vi "GeoData.vi"() -> ()   [LabVIEW 2017] (continued)
Davison County\tH1\n57235\t46037\tFlorence\tSD\tDay County\tH1\n57239\t46037\tGrenville\tSD\tDay County\tH1\n57434\t46037\tConde\tSD\tDay County\tH1\n57273\t46037\tWaubay\tSD\tDay County\tH1\n57454\t46037\tLangford\tSD\tDay County\tH1\n57232\t46037\tEden\tSD\tDay County\tH1\n57272\t46037\tWallace\tSD\tDay County\tH1\n57422\t46037\tAndover\tSD\tDay County\tH1\n57274\t46037\tWebster\tSD\tDay County\tH1\n57445\t46037\tGroton\tSD\tDay County\tH1\n57219\t46037\tBristol\tSD\tDay County\tH1\n57468\t46037\tPierpont\tSD\tDay County\tH1\n57256\t46037\tOrtley\tSD\tDay County\tH1\n57261\t46037\tRoslyn\tSD\tDay County\tH1\n57234\t46039\tEstelline\tSD\tDeuel County\tH1\n57238\t46039\tGoodwin\tSD\tDeuel County\tH1\n57268\t46039\tToronto\tSD\tDeuel County\tH1\n57265\t46039\tStrandburg\tSD\tDeuel County\tH1\n57213\t46039\tAstoria\tSD\tDeuel County\tH1\n57226\t46039\tClear lake\tSD\tDeuel County\tH1\n57223\t46039\tCastlewood\tSD\tDeuel County\tH1\n57237\t46039\tGary\tSD\tDeuel County\tH1\n57259\t46039\tRevillo\tSD\tDeuel County\tH1\n57218\t46039\tBrandt\tSD\tDeuel County\tH1\n57652\t46041\tRidgeview\tSD\tDewey County\tH1\n57657\t46041\tTrail city\tSD\tDewey County\tH1\n57633\t46041\tIsabel\tSD\tDewey County\tH1\n57630\t46041\tGlencross\tSD\tDewey County\tH1\n57636\t46041\tLantry\tSD\tDewey County\tH1\n57656\t46041\tTimber lake\tSD\tDewey County\tH1\n57625\t46041\tEagle butte\tSD\tDewey County\tH1\n57661\t46041\tWhitehorse\tSD\tDewey County\tH1\n57344\t46043\tHarrison\tSD\tDouglas County\tH1\n57313\t46043\tArmour\tSD\tDouglas County\tH1\n57369\t46043\tPlatte\tSD\tDouglas County\tH1\n57328\t46043\tCorsica\tSD\tDouglas County\tH1\n57331\t46043\tDimock\tSD\tDouglas County\tH1\n57375\t46043\tStickney\tSD\tDouglas County\tH1\n57330\t46043\tDelmont\tSD\tDouglas County\tH1\n57364\t46043\tNew holland\tSD\tDouglas County\tH1\n57366\t46043\tParkston\tSD\tDouglas County\tH1\n57342\t46043\tGeddes\tSD\tDouglas County\tH1\n57451\t46045\tIpswich\tSD\tEdmunds County\tH1\n57428\t46045\tBowdle\tSD\tEdmunds County\tH1\n57460\t46045\tMansfield\tSD\tEdmunds County\tH1\n57471\t46045\tRoscoe\tSD\tEdmunds County\tH1\n57481\t46045\tWestport\tSD\tEdmunds County\tH1\n57448\t46045\tHosmer\tSD\tEdmunds County\tH1\n57435\t46045\tCresbard\tSD\tEdmunds County\tH1\n57475\t46045\tTolstoy\tSD\tEdmunds County\tH1\n57456\t46045\tLeola\tSD\tEdmunds County\tH1\n57466\t46045\tOnaka\tSD\tEdmunds County\tH1\n57722\t46047\tBuffalo gap\tSD\tFall River County\tH1\n57747\t46047\tHot springs\tSD\tFall River County\tH1\n57782\t46047\tSmithwick\tSD\tFall River County\tH1\n57735\t46047\tEdgemont\tSD\tFall River County\tH1\n57766\t46047\tOral\tSD\tFall River County\tH1\n57763\t46047\tOelrichs\tSD\tFall River County\tH1\n57460\t46049\tMansfield\tSD\tFaulk County\tH1\n57438\t46049\tFaulkton\tSD\tFaulk County\tH1\n57424\t46049\tAshton\tSD\tFaulk County\tH1\n57469\t46049\tRedfield\tSD\tFaulk County\tH1\n57470\t46049\tRockham\tSD\tFaulk County\tH1\n57435\t46049\tCresbard\tSD\tFaulk County\tH1\n57467\t46049\tOrient\tSD\tFaulk County\tH1\n57473\t46049\tSeneca\tSD\tFaulk County\tH1\n57465\t46049\tNorthville\tSD\tFaulk County\tH1\n57345\t46049\tHighmore\tSD\tFaulk County\tH1\n57466\t46049\tOnaka\tSD\tFaulk County\tH1\n57252\t46051\tMilbank\tSD\tGrant County\tH1\n57279\t46051\tWilmot\tSD\tGrant County\tH1\n57216\t46051\tBig stone city\tSD\tGrant County\tH1\n57273\t46051\tWaubay\tSD\tGrant County\tH1\n57227\t46051\tCorona\tSD\tGrant County\tH1\n57238\t46051\tGoodwin\tSD\tGrant County\tH1\n57263\t46051\tSouth shore\tSD\tGrant County\tH1\n57265\t46051\tStrandburg\tSD\tGrant County\tH1\n57266\t46051\tSummit\tSD\tGrant County\tH1\n57246\t46051\tLabolt\tSD\tGrant County\tH1\n57269\t46051\tTwin brooks\tSD\tGrant County\tH1\n57251\t46051\tMarvin\tSD\tGrant County\tH1\n57264\t46051\tStockholm\tSD\tGrant County\tH1\n57256\t46051\tOrtley\tSD\tGrant County\tH1\n57259\t46051\tRevillo\tSD\tGrant County\tH1\n57529\t46053\tDallas\tSD\tGregory County\tH1\n57538\t46053\tHerrick\tSD\tGregory County\tH1\n57317\t46053\tBonesteel\tSD\tGregory County\tH1\n57335\t46053\tFairfax\tSD\tGregory County\tH1\n57523\t46053\tBurke\tSD\tGregory County\tH1\n57571\t46053\tSaint charles\tSD\tGregory County\tH1\n57533\t46053\tGregory\tSD\tGregory County\tH1\n57552\t46055\tMidland\tSD\tHaakon County\tH1\n57567\t46055\tPhilip\tSD\tHaakon County\tH1\n57775\t46055\tQuinn\tSD\tHaakon County\tH1\n57543\t46055\tKadoka\tSD\tHaakon County\tH1\n57553\t46055\tMilesville\tSD\tHaakon County\tH1\n57234\t46057\tEstelline\tSD\tHamlin County\tH1\n57233\t46057\tErwin\tSD\tHamlin County\tH1\n57221\t46057\tBryant\tSD\tHamlin County\tH1\n57238\t46057\tGoodwin\tSD\tHamlin County\tH1\n57212\t46057\tArlington\tSD\tHamlin County\tH1\n57271\t46057\tVienna\tSD\tHamlin County\tH1\n57242\t46057\tHazel\tSD\tHamlin County\tH1\n57241\t46057\tHayti\tSD\tHamlin County\tH1\n57248\t46057\tLake norden\tSD\tHamlin County\tH1\n57226\t46057\tClear lake\tSD\tHamlin County\tH1\n57201\t46057\tWatertown\tSD\tHamlin County\tH1\n57243\t46057\tHenry\tSD\tHamlin County\tH1\n57223\t46057\tCastlewood\tSD\tHamlin County\tH1\n57476\t46059\tTulare\tSD\tHand County\tH1\n57469\t46059\tRedfield\tSD\tHand County\tH1\n57470\t46059\tRockham\tSD\tHand County\tH1\n57362\t46059\tMiller\tSD\tHand County\tH1\n57381\t46059\tWessington\tSD\tHand County\tH1\n57373\t46059\tSaint lawrence\tSD\tHand County\tH1\n57371\t46059\tRee heights\tSD\tHand County\tH1\n57467\t46059\tOrient\tSD\tHand County\tH1\n57382\t46059\tWessington springs\tSD\tHand County\tH1\n57345\t46059\tHighmore\tSD\tHand County\tH1\n57319\t46061\tBridgewater\tSD\tHanson County\tH1\n57340\t46061\tFulton\tSD\tHanson County\tH1\n57311\t46061\tAlexandria\tSD\tHanson County\tH1\n57334\t46061\tEthan\tSD\tHanson County\tH1\n57374\t46061\tSpencer\tSD\tHanson County\tH1\n57301\t46061\tMitchell\tSD\tHanson County\tH1\n57321\t46061\tCanova\tSD\tHanson County\tH1\n57332\t46061\tEmery\tSD\tHanson County\tH1\n57366\t46061\tParkston\tSD\tHanson County\tH1\n57760\t46063\tNewell\tSD\tHarding County\tH1\n57650\t46063\tRalph\tSD\tHarding County\tH1\n57755\t46063\tLudlow\tSD\tHarding County\tH1\n57651\t46063\tReva\tSD\tHarding County\tH1\n57717\t46063\tBelle fourche\tSD\tHarding County\tH1\n57720\t46063\tBuffalo\tSD\tHarding County\tH1\n57724\t46063\tCamp crook\tSD\tHarding County\tH1\n57649\t46063\tPrairie city\tSD\tHarding County\tH1\n57776\t46063\tRedig\tSD\tHarding County\tH1\n57501\t46065\tPierre\tSD\tHughes County\tH1\n57564\t46065\tOnida\tSD\tHughes County\tH1\n57536\t46065\tHarrold\tSD\tHughes County\tH1\n57522\t46065\tBlunt\tSD\tHughes County\tH1\n57319\t46067\tBridgewater\tSD\tHutchinson County\tH1\n57043\t46067\tMarion\tSD\tHutchinson County\tH1\n57354\t46067\tKaylor\tSD\tHutchinson County\tH1\n57059\t46067\tScotland\tSD\tHutchinson County\tH1\n57311\t46067\tAlexandria\tSD\tHutchinson County\tH1\n57334\t46067\tEthan\tSD\tHutchinson County\tH1\n57331\t46067\tDimock\tSD\tHutchinson County\tH1\n57052\t46067\tOlivet\tSD\tHutchinson County\tH1\n57029\t46067\tFreeman\tSD\tHutchinson County\tH1\n57330\t46067\tDelmont\tSD\tHutchinson County\tH1\n57045\t46067\tMenno\tSD\tHutchinson County\tH1\n57332\t46067\tEmery\tSD\tHutchinson County\tH1\n57376\t46067\tTripp\tSD\tHutchinson County\tH1\n57366\t46067\tParkston\tSD\tHutchinson County\tH1\n57540\t46069\tHolabird\tSD\tHyde County\tH1\n57346\t46069\tStephan\tSD\tHyde County\tH1\n57564\t46069\tOnida\tSD\tHyde County\tH1\n57345\t46069\tHighmore\tSD\tHyde County\tH1\n57536\t46069\tHarrold\tSD\tHyde County\tH1\n57577\t46071\tWanblee\tSD\tJackson County\tH1\n57567\t46071\tPhilip\tSD\tJackson County\tH1\n57521\t46071\tBelvidere\tSD\tJackson County\tH1\n57543\t46071\tKadoka\tSD\tJackson County\tH1\n57750\t46071\tInterior\tSD\tJackson County\tH1\n57547\t46071\tLong valley\tSD\tJackson County\tH1\n57312\t46073\tAlpena\tSD\tJerauld County\tH1\n57385\t46073\tWoonsocket\tSD\tJerauld County\tH1\n57382\t46073\tWessington springs\tSD\tJerauld County\tH1\n57355\t46073\tKimball\tSD\tJerauld County\tH1\n57531\t46075\tDraper\tSD\tJones County\tH1\n57559\t46075\tMurdo\tSD\tJones County\tH1\n57562\t46075\tOkaton\tSD\tJones County\tH1\n57231\t46077\tDe smet\tSD\tKingsbury County\tH1\n57233\t46077\tErwin\tSD\tKingsbury County\tH1\n57221\t46077\tBryant\tSD\tKingsbury County\tH1\n57051\t46077\tOldham\tSD\tKingsbury County\tH1\n57212\t46077\tArlington\tSD\tKingsbury County\tH1\n57248\t46077\tLake norden\tSD\tKingsbury County\tH1\n57054\t46077\tRamona\tSD\tKingsbury County\tH1\n57323\t46077\tCarthage\tSD\tKingsbury County\tH1\n57386\t46077\tYale\tSD\tKingsbury County\tH1\n57249\t46077\tLake preston\tSD\tKingsbury County\tH1\n57353\t46077\tIroquois\tSD\tKingsbury County\tH1\n57214\t46077\tBadger\tSD\tKingsbury County\tH1\n57048\t46079\tMontrose\tSD\tLake County\tH1\n57058\t46079\tSalem\tSD\tLake County\tH1\n57042\t46079\tMadison\tSD\tLake County\tH1\n57017\t46079\tColman\tSD\tLake County\tH1\n57051\t46079\tOldham\tSD\tLake County\tH1\n57212\t46079\tArlington\tSD\tLake County\tH1\n57076\t46079\tWinfred\tSD\tLake County\tH1\n57054\t46079\tRamona\tSD\tLake County\tH1\n57018\t46079\tColton\tSD\tLake County\tH1\n57016\t46079\tChester\tSD\tLake County\tH1\n57022\t46079\tDell rapids\tSD\tLake County\tH1\n57075\t46079\tWentworth\tSD\tLake County\tH1\n57057\t46079\tRutland\tSD\tLake County\tH1\n57071\t46079\tVolga\tSD\tLake County\tH1\n57050\t46079\tNunda\tSD\tLake County\tH1\n57779\t46081\tSaint onge\tSD\tLawrence County\tH1\n57785\t46081\tSturgis\tSD\tLawrence County\tH1\n57759\t46081\tNemo\tSD\tLawrence County\tH1\n57783\t46081\tSpearfish\tSD\tLawrence County\tH1\n57754\t46081\tLead\tSD\tLawrence County\tH1\n57717\t46081\tBelle fourche\tSD\tLawrence County\tH1\n57793\t46081\tWhitewood\tSD\tLawrence County\tH1\n57732\t46081\tDeadwood\tSD\tLawrence County\tH1\n57799\t46081\tSpearfish\tSD\tLawrence County\tH1\n57032\t46083\tHarrisburg\tSD\tLincoln County\tH1\n57021\t46083\tDavis\tSD\tLincoln County\tH1\n57106\t46083\tSioux falls\tSD\tLincoln County\tH1\n57014\t46083\tCenterville\tSD\tLincoln County\tH1\n57027\t46083\tFairview\tSD\tLincoln County\tH1\n57064\t46083\tTea\tSD\tLincoln County\tH1\n57108\t46083\tSioux falls\tSD\tLincoln County\tH1\n57034\t46083\tHudson\tSD\tLincoln County\tH1\n57039\t46083\tLennox\tSD\tLincoln County\tH1\n57077\t46083\tWorthing\tSD\tLincoln County\tH1\n57013\t46083\tCanton\tSD\tLincoln County\tH1\n57004\t46083\tBeresford\tSD\tLincoln County\tH1\n57104\t46083\tSioux falls\tSD\tLincoln County\tH1\n57001\t46083\tAlcester\tSD\tLincoln County\tH1\n57576\t46085\tVivian\tSD\tLyman County\tH1\n57568\t46085\tPresho\tSD\tLyman County\tH1\n57544\t46085\tKennebec\tSD\tLyman County\tH1\n57569\t46085\tReliance\tSD\tLyman County\tH1\n57548\t46085\tLower brule\tSD\tLyman County\tH1\n57533\t46085\tGregory\tSD\tLyman County\tH1\n57534\t46085\tHamill\tSD\tLyman County\tH1\n57365\t46085\tOacoma\tSD\tLyman County\tH1\n57048\t46087\tMontrose\tSD\tMcCook County\tH1\n57053\t46087\tParker\tSD\tMcCook County\tH1\n57058\t46087\tSalem\tSD\tMcCook County\tH1\n57042\t46087\tMadison\tSD\tMcCook County\tH1\n57319\t46087\tBridgewater\tSD\tMcCook County\tH1\n57043\t46087\tMarion\tSD\tMcCook County\tH1\n57012\t46087\tCanistota\tSD\tMcCook County\tH1\n57047\t46087\tMonroe\tSD\tMcCook County\tH1\n57374\t46087\tSpencer\tSD\tMcCook County\tH1\n57035\t46087\tHumboldt\tSD\tMcCook County\tH1\n57321\t46087\tCanova\tSD\tMcCook County\tH1\n57332\t46087\tEmery\tSD\tMcCook County\tH1\n57428\t46089\tBowdle\tSD\tMcPherson County\tH1\n57471\t46089\tRoscoe\tSD\tMcPherson County\tH1\n57481\t46089\tWestport\tSD\tMcPherson County\tH1\n57437\t46089\tEureka\tSD\tMcPherson County\tH1\n57448\t46089\tHosmer\tSD\tMcPherson County\tH1\n57456\t46089\tLeola\tSD\tMcPherson County\tH1\n57457\t46089\tLong lake\tSD\tMcPherson County\tH1\n57247\t46091\tLake city\tSD\tMarshall County\tH1\n57454\t46091\tLangford\tSD\tMarshall County\tH1\n57432\t46091\tClaremont\tSD\tMarshall County\tH1\n57232\t46091\tEden\tSD\tMarshall County\tH1\n57430\t46091\tBritton\tSD\tMarshall County\tH1\n57262\t46091\tSisseton\tSD\tMarshall County\tH1\n57270\t46091\tVeblen\tSD\tMarshall County\tH1\n57421\t46091\tAmherst\tSD\tMarshall County\tH1\n57787\t46093\tUnion center\tSD\tMeade County\tH1\n57767\t46093\tOwanka\tSD\tMeade County\tH1\n57788\t46093\tVale\tSD\tMeade County\tH1\n57785\t46093\tSturgis\tSD\tMeade County\tH1\n57748\t46093\tHowes\tSD\tMeade County\tH1\n57701\t46093\tRapid city\tSD\tMeade County\tH1\n57702\t46093\tRapid city\tSD\tMeade County\tH1\n57718\t46093\tBlack hawk\tSD\tMeade County\tH1\n57791\t46093\tWasta\tSD\tMeade County\tH1\n57761\t46093\tNew underwood\tSD\tMeade County\tH1\n57758\t46093\tMud butte\tSD\tMeade County\tH1\n57737\t46093\tEnning\tSD\tMeade County\tH1\n57719\t46093\tBox elder\tSD\tMeade County\tH1\n57769\t46093\tPiedmont\tSD\tMeade County\tH1\n57626\t46093\tFaith\tSD\tMeade County\tH1\n57793\t46093\tWhitewood\tSD\tMeade County\tH1\n57792\t46093\tWhite owl\tSD\tMeade County\tH1\n57706\t46093\tEllsworth afb\tSD\tMeade County\tH1\n57741\t46093\tFort meade\tSD\tMeade County\tH1\n57579\t46095\tWhite river\tSD\tMellette County\tH1\n57560\t46095\tNorris\tSD\tMellette County\tH1\n57585\t46095\tWood\tSD\tMellette County\tH1\n57058\t46097\tSalem\tSD\tMiner County\tH1\n57051\t46097\tOldham\tSD\tMiner County\tH1\n57337\t46097\tFedora\tSD\tMiner County\tH1\n57340\t46097\tFulton\tSD\tMiner County\tH1\n57076\t46097\tWinfred\tSD\tMiner County\tH1\n57054\t46097\tRamona\tSD\tMiner County\tH1\n57323\t46097\tCarthage\tSD\tMiner County\tH1\n57349\t46097\tHoward\tSD\tMiner County\tH1\n57321\t46097\tCanova\tSD\tMiner County\tH1\n57048\t46099\tMontrose\tSD\tMinnehaha County\tH1\n57053\t46099\tParker\tSD\tMinnehaha County\tH1\n57103\t46099\tSioux falls\tSD\tMinnehaha County\tH1\n57005\t46099\tBrandon\tSD\tMinnehaha County\tH1\n57042\t46099\tMadison\tSD\tMinnehaha County\tH1\n57106\t46099\tSioux falls\tSD\tMinnehaha County\tH1\n57068\t46099\tValley springs\tSD\tMinnehaha County\tH1\n57041\t46099\tLyons\tSD\tMinnehaha County\tH1\n57064\t46099\tTea\tSD\tMinnehaha County\tH1\n57108\t46099\tSioux falls\tSD\tMinnehaha County\tH1\n57110\t46099\tSioux falls\tSD\tMinnehaha County\tH1\n57118\t46099\tSioux falls\tSD\tMinnehaha County\tH1\n57109\t46099\tSioux falls\tSD\tMinnehaha County\tH1\n57015\t46099\tChancellor\tSD\tMinnehaha County\tH1\n57055\t46099\tRenner\tSD\tMinnehaha County\tH1\n57101\t46099\tSioux falls\tSD\tMinnehaha County\tH1\n57018\t46099\tColton\tSD\tMinnehaha County\tH1\n57016\t46099\tChester\tSD\tMinnehaha County\tH1\n57105\t46099\tSioux falls\tSD\tMinnehaha County\tH1\n57107\t46099\tSioux falls\tSD\tMinnehaha County\tH1\n57035\t46099\tHumboldt\tSD\tMinnehaha County\tH1\n57022\t46099\tDell rapids\tSD\tMinnehaha County\tH1\n57020\t46099\tCrooks\tSD\tMinnehaha County\tH1\n57198\t46099\tSioux falls\tSD\tMinnehaha County\tH1\n57193\t46099\tSioux falls\tSD\tMinnehaha County\tH1\n57030\t46099\tGarretson\tSD\tMinnehaha County\tH1\n57186\t46099\tSioux falls\tSD\tMinnehaha County\tH1\n57197\t46099\tSioux falls\tSD\tMinnehaha County\tH1\n57104\t46099\tSioux falls\tSD\tMinnehaha County\tH1\n57033\t46099\tHartford\tSD\tMinnehaha County\tH1\n57003\t46099\tBaltic\tSD\tMinnehaha County\tH1\n57017\t46101\tColman\tSD\tMoody County\tH1\n57026\t46101\tElkton\tSD\tMoody County\tH1\n57002\t46101\tAurora\tSD\tMoody County\tH1\n57024\t46101\tEgan\tSD\tMoody County\tH1\n57006\t46101\tBrookings\tSD\tMoody County\tH1\n57065\t46101\tTrent\tSD\tMoody County\tH1\n57022\t46101\tDell rapids\tSD\tMoody County\tH1\n57075\t46101\tWentworth\tSD\tMoody County\tH1\n57057\t46101\tRutland\tSD\tMoody County\tH1\n57071\t46101\tVolga\tSD\tMoody County\tH1\n57028\t46101\tFlandreau\tSD\tMoody County\tH1\n57703\t46103\tRapid city\tSD\tPennington County\tH1\n57725\t46103\tCaputa\tSD\tPennington County\tH1\n57767\t46103\tOwanka\tSD\tPennington County\tH1\n57701\t46103\tRapid city\tSD\tPennington County\tH1\n57702\t46103\tRapid city\tSD\tPennington County\tH1\n57718\t46103\tBlack hawk\tSD\tPennington County\tH1\n57791\t46103\tWasta\tSD\tPennington County\tH1\n57761\t46103\tNew underwood\tSD\tPennington County\tH1\n57754\t46103\tLead\tSD\tPennington County\tH1\n57744\t46103\tHermosa\tSD\tPennington County\tH1\n57719\t46103\tBox elder\tSD\tPennington County\tH1\n57567\t46103\tPhilip\tSD\tPennington County\tH1\n57780\t46103\tScenic\tSD\tPennington County\tH1\n57730\t46103\tCuster\tSD\tPennington County\tH1\n57775\t46103\tQuinn\tSD\tPennington County\tH1\n57790\t46103\tWall\tSD\tPennington County\tH1\n57750\t46103\tInterior\tSD\tPennington County\tH1\n57732\t46103\tDeadwood\tSD\tPennington County\tH1\n57745\t46103\tHill city\tSD\tPennington County\tH1\n57751\t46103\tKeystone\tSD\tPennington County\tH1\n57709\t46103\tRapid city\tSD\tPennington County\tH1\n57706\t46103\tEllsworth afb\tSD\tPennington County\tH1\n57640\t46105\tLodgepole\tSD\tPerkins County\tH1\n57651\t46105\tReva\tSD\tPerkins County\tH1\n57758\t46105\tMud butte\tSD\tPerkins County\tH1\n57620\t46105\tBison\tSD\tPerkins County\tH1\n57638\t46105\tLemmon\tSD\tPerkins County\tH1\n57626\t46105\tFaith\tSD\tPerkins County\tH1\n57644\t46105\tMeadow\tSD\tPerkins County\tH1\n57649\t46105\tPrairie city\tSD\tPerkins County\tH1\n57450\t46107\tHoven\tSD\tPotter County\tH1\n57442\t46107\tGettysburg\tSD\tPotter County\tH1\n57475\t46107\tTolstoy\tSD\tPotter County\tH1\n57473\t46107\tSeneca\tSD\tPotter County\tH1\n57455\t46107\tLebanon\tSD\tPotter County\tH1\n57252\t46109\tMilbank\tSD\tRoberts County\tH1\n57279\t46109\tWilmot\tSD\tRoberts County\tH1\n57216\t46109\tBig stone city\tSD\tRoberts County\tH1\n57273\t46109\tWaubay\tSD\tRoberts County\tH1\n57227\t46109\tCorona\tSD\tRoberts County\tH1\n57224\t46109\tClaire city\tSD\tRoberts County\tH1\n57257\t46109\tPeever\tSD\tRoberts County\tH1\n57266\t46109\tSummit\tSD\tRoberts County\tH1\n57262\t46109\tSisseton\tSD\tRoberts County\tH1\n57270\t46109\tVeblen\tSD\tRoberts County\tH1\n57255\t46109\tNew effington\tSD\tRoberts County\tH1\n57256\t46109\tOrtley\tSD\tRoberts County\tH1\n57260\t46109\tRosholt\tSD\tRoberts County\tH1\n57312\t46111\tAlpena\tSD\tSanborn County\tH1\n57358\t46111\tLane\tSD\tSanborn County\tH1\n57337\t46111\tFedora\tSD\tSanborn County\tH1\n57363\t46111\tMount vernon\tSD\tSanborn County\tH1\n57385\t46111\tWoonsocket\tSD\tSanborn County\tH1\n57314\t46111\tArtesian\tSD\tSanborn County\tH1\n57323\t46111\tCarthage\tSD\tSanborn County\tH1\n57350\t46111\tHuron\tSD\tSanborn County\tH1\n57359\t46111\tLetcher\tSD\tSanborn County\tH1\n57460\t46115\tMansfield\tSD\tSpink County\tH1\n57434\t46115\tConde\tSD\tSpink County\tH1\n57477\t46115\tTurton\tSD\tSpink County\tH1\n57476\t46115\tTulare\tSD\tSpink County\tH1\n57440\t46115\tFrankfort\tSD\tSpink County\tH1\n57424\t46115\tAshton\tSD\tSpink County\tH1\n57469\t46115\tRedfield\tSD\tSpink County\tH1\n57429\t46115\tBrentford\tSD\tSpink County\tH1\n57322\t46115\tCarpenter\tSD\tSpink County\tH1\n57461\t46115\tMellette\tSD\tSpink County\tH1\n57465\t46115\tNorthville\tSD\tSpink County\tH1\n57474\t46115\tStratford\tSD\tSpink County\tH1\n57348\t46115\tHitchcock\tSD\tSpink County\tH1\n57436\t46115\tDoland\tSD\tSpink County\tH1\n57258\t46115\tRaymond\tSD\tSpink County\tH1\n57532\t46117\tFort pierre\tSD\tStanley County\tH1\n57552\t46117\tMidland\tSD\tStanley County\tH1\n57537\t46117\tHayes\tSD\tStanley County\tH1\n57442\t46119\tGettysburg\tSD\tSully County\tH1\n57501\t46119\tPierre\tSD\tSully County\tH1\n57520\t46119\tAgar\tSD\tSully County\tH1\n57564\t46119\tOnida\tSD\tSully County\tH1\n57536\t46119\tHarrold\tSD\tSully County\tH1\n57522\t46119\tBlunt\tSD\tSully County\tH1\n57580\t46121\tWinner\tSD\tTodd County\tH1\n57572\t46121\tSaint francis\tSD\tTodd County\tH1\n57570\t46121\tRosebud\tSD\tTodd County\tH1\n57566\t46121\tParmelee\tSD\tTodd County\tH1\n57555\t46121\tMission\tSD\tTodd County\tH1\n57563\t46121\tOkreek\tSD\tTodd County\tH1\n57580\t46123\tWinner\tSD\tTripp County\tH1\n57529\t46123\tDallas\tSD\tTripp County\tH1\n57584\t46123\tWitten\tSD\tTripp County\tH1\n57528\t46123\tColome\tSD\tTripp County\tH1\n57533\t46123\tGregory\tSD\tTripp County\tH1\n57534\t46123\tHamill\tSD\tTripp County\tH1\n57541\t46123\tIdeal\tSD\tTripp County\tH1\n57053\t46125\tParker\tSD\tTurner County\tH1\n57073\t46125\tWakonda\tSD\tTurner County\tH1\n57070\t46125\tViborg\tSD\tTurner County\tH1\n57021\t46125\tDavis\tSD\tTurner County\tH1\n57319\t46125\tBridgewater\tSD\tTurner County\tH1\n57043\t46125\tMarion\tSD\tTurner County\tH1\n57014\t46125\tCenterville\tSD\tTurner County\tH1\n57047\t46125\tMonroe\tSD\tTurner County\tH1\n57064\t46125\tTea\tSD\tTurner County\tH1\n57015\t46125\tChancellor\tSD\tTurner County\tH1\n57039\t46125\tLennox\tSD\tTurner County\tH1\n57029\t46125\tFreeman\tSD\tTurner County\tH1\n57037\t46125\tIrene\tSD\tTurner County\tH1\n57045\t46125\tMenno\tSD\tTurner County\tH1\n57036\t46125\tHurley\tSD\tTurner County\tH1\n57025\t46127\tElk point\tSD\tUnion County\tH1\n57010\t46127\tBurbank\tSD\tUnion County\tH1\n57049\t46127\tNorth sioux city\tSD\tUnion County\tH1\n57034\t46127\tHudson\tSD\tUnion County\tH1\n57038\t46127\tJefferson\tSD\tUnion County\tH1\n57004\t46127\tBeresford\tSD\tUnion County\tH1\n57001\t46127\tAlcester\tSD\tUnion County\tH1\n57428\t46129\tBowdle\tSD\tWalworth County\tH1\n57450\t46129\tHoven\tSD\tWalworth County\tH1\n57631\t46129\tGlenham\tSD\tWalworth County\tH1\n57601\t46129\tMobridge\tSD\tWalworth County\tH1\n57472\t46129\tSelby\tSD\tWalworth County\tH1\n57420\t46129\tAkaska\tSD\tWalworth County\tH1\n57452\t46129\tJava\tSD\tWalworth County\tH1\n57070\t46135\tViborg\tSD\tYankton County\tH1\n57063\t46135\tTabor\tSD\tYankton County\tH1\n57059\t46135\tScotland\tSD\tYankton County\tH1\n57072\t46135\tVolin\tSD\tYankton County\tH1\n57037\t46135\tIrene\tSD\tYankton County\tH1\n57045\t46135\tMenno\tSD\tYankton County\tH1\n57031\t46135\tGayville\tSD\tYankton County\tH1\n57046\t46135\tMission hill\tSD\tYankton County\tH1\n57078\t46135\tYankton\tSD\tYankton County\tH1\n57040\t46135\tLesterville\tSD\tYankton County\tH1\n57067\t46135\tUtica\tSD\tYankton County\tH1\n57623\t46137\tDupree\tSD\tZiebach County\tH1\n57622\t46137\tCherry creek\tSD\tZiebach County\tH1\n37938\t47001\tKnoxville\tTN\tAnderson County\tH1\n37717\t47001\tClinton\tTN\tAnderson County\tH1\n37705\t47001\tAndersonville\tTN\tAnderson County\tH1\n37754\t47001\tHeiskell\tTN\tAnderson County\tH1\n37828\t47001\tNorris\tTN\tAnderson County\tH1\n37840\t47001\tOliver springs\tTN\tAnderson County\tH1\n37849\t47001\tPowell\tTN\tAnderson County\tH1\n37769\t47001\tRocky top\tTN\tAnderson County\tH1\n37716\t47001\tClinton\tTN\tAnderson County\tH1\n37931\t47001\tKnoxville\tTN\tAnderson County\tH1\n37830\t47001\tOak ridge\tTN\tAnderson County\tH1\n37710\t47001\tBriceville\tTN\tAnderson County\tH1\n37831\t47001\tOak ridge\tTN\tAnderson County\tH1\n37060\t47003\tEagleville\tTN\tBedford County\tH1\n37153\t47003\tRockvale\tTN\tBedford County\tH1\n37334\t47003\tFayetteville\tTN\tBedford County\tH1\n37034\t47003\tChapel hill\tTN\tBedford County\tH1\n37020\t47003\tBell buckle\tTN\tBedford County\tH1\n37183\t47003\tWartrace\tTN\tBedford County\tH1\n37144\t47003\tPetersburg\tTN\tBedford County\tH1\n37388\t47003\tTullahoma\tTN\tBedford County\tH1\n37091\t47003\tLewisburg\tTN\tBedford County\tH1\n37018\t47003\tBeechgrove\tTN\tBedford County\tH1\n37180\t47003\tUnionville\tTN\tBedford County\tH1\n37161\t47003\tShelbyville\tTN\tBedford County\tH1\n37160\t47003\tShelbyville\tTN\tBedford County\tH1\n37360\t47003\tNormandy\tTN\tBedford County\tH1\n38318\t47005\tBuena vista\tTN\tBenton County\tH1\n38317\t47005\tBruceton\tTN\tBenton County\tH1\n38320\t47005\tCamden\tTN\tBenton County\tH1\n38341\t47005\tHolladay\tTN\tBenton County\tH1\n38387\t47005\tWestport\tTN\tBenton County\tH1\n38221\t47005\tBig sandy\tTN\tBenton County\tH1\n38333\t47005\tEva\tTN\tBenton County\tH1\n38380\t47005\tSugar tree\tTN\tBenton County\tH1\n37379\t47007\tSoddy daisy\tTN\tBledsoe County\tH1\n37381\t47007\tSpring city\tTN\tBledsoe County\tH1\n37338\t47007\tGraysville\tTN\tBledsoe County\tH1\n37367\t47007\tPikeville\tTN\tBledsoe County\tH1\n37332\t47007\tEvensville\tTN\tBledsoe County\tH1\n38572\t47007\tCrossville\tTN\tBledsoe County\tH1\n37327\t47007\tDunlap\tTN\tBledsoe County\tH1\n37337\t47007\tGrandview\tTN\tBledsoe County\tH1\n37321\t47007\tDayton\tTN\tBledsoe County\tH1\n37865\t47009\tSeymour\tTN\tBlount County\tH1\n37802\t47009\tMaryville\tTN\tBlount County\tH1\n37737\t47009\tFriendsville\tTN\tBlount County\tH1\n37886\t47009\tWalland\tTN\tBlount County\tH1\n37804\t47009\tMaryville\tTN\tBlount County\tH1\n37882\t47009\tTownsend\tTN\tBlount County\tH1\n37772\t47009\tLenoir city\tTN\tBlount County\tH1\n37801\t47009\tMaryville\tTN\tBlount County\tH1\n37878\t47009\tTallassee\tTN\tBlount County\tH1\n37920\t47009\tKnoxville\tTN\tBlount County\tH1\n37853\t47009\tRockford\tTN\tBlount County\tH1\n37803\t47009\tMaryville\tTN\tBlount County\tH1\n37777\t47009\tLouisville\tTN\tBlount County\tH1\n37701\t47009\tAlcoa\tTN\tBlount County\tH1\n37742\t47009\tGreenback\tTN\tBlount County\tH1\n37353\t47011\tMc donald\tTN\tBradley County\tH1\n37311\t47011\tCleveland\tTN\tBradley County\tH1\n37362\t47011\tOld fort\tTN\tBradley County\tH1\n37310\t47011\tCharleston\tTN\tBradley County\tH1\n37364\t47011\tCleveland\tTN\tBradley County\tH1\n37312\t47011\tCleveland\tTN\tBradley County\tH1\n37323\t47011\tCleveland\tTN\tBradley County\tH1\n37336\t47011\tGeorgetown\tTN\tBradley County\tH1\n37320\t47011\tCleveland\tTN\tBradley County\tH1\n37756\t47013\tHuntsville\tTN\tCampbell County\tH1\n37847\t47013\tPioneer\tTN\tCampbell County\tH1\n37714\t47013\tCaryville\tTN\tCampbell County\tH1\n37769\t47013\tRocky top\tTN\tCampbell County\tH1\n37766\t47013\tLa follette\tTN\tCampbell County\tH1\n37762\t47013\tJellico\tTN\tCampbell County\tH1\n37757\t47013\tJacksboro\tTN\tCampbell County\tH1\n37715\t47013\tClairfield\tTN\tCampbell County\tH1\n37870\t47013\tSpeedwell\tTN\tCampbell County\tH1\n37819\t47013\tNewcomb\tTN\tCampbell County\tH1\n37729\t47013\tDuff\tTN\tCampbell County\tH1\n37118\t47015\tMilton\tTN\tCannon County\tH1\n37166\t47015\tSmithville\tTN\tCannon County\tH1\n37357\t47015\tMorrison\tTN\tCannon County\tH1\n37016\t47015\tAuburntown\tTN\tCannon County\tH1\n37037\t47015\tChristiana\tTN\tCannon County\tH1\n37026\t47015\tBradyville\tTN\tCannon County\tH1\n37190\t47015\tWoodbury\tTN\tCannon County\tH1\n37149\t47015\tReadyville\tTN\tCannon County\tH1\n37095\t47015\tLiberty\tTN\tCannon County\tH1\n37018\t47015\tBeechgrove\tTN\tCannon County\tH1\n37110\t47015\tMcminnville\tTN\tCannon County\tH1\n38220\t47017\tAtwood\tTN\tCarroll County\tH1\n38201\t47017\tMc kenzie\tTN\tCarroll County\tH1\n38344\t47017\tHuntingdon\tTN\tCarroll County\tH1\n38358\t47017\tMilan\tTN\tCarroll County\tH1\n38318\t47017\tBuena vista\tTN\tCarroll County\tH1\n38317\t47017\tBruceton\tTN\tCarroll County\tH1\n38390\t47017\tYuma\tTN\tCarroll County\tH1\n38320\t47017\tCamden\tTN\tCarroll County\tH1\n38341\t47017\tHolladay\tTN\tCarroll County\tH1\n38324\t47017\tClarksburg\tTN\tCarroll County\tH1\n38235\t47017\tMc lemoresville\tTN\tCarroll County\tH1\n38305\t47017\tJackson\tTN\tCarroll County\tH1\n38321\t47017\tCedar grove\tTN\tCarroll County\tH1\n38348\t47017\tLavinia\tTN\tCarroll County\tH1\n38387\t47017\tWestport\tTN\tCarroll County\tH1\n38388\t47017\tWildersville\tTN\tCarroll County\tH1\n38258\t47017\tTrezevant\tTN\tCarroll County\tH1\n38342\t47017\tHollow rock\tTN\tCarroll County\tH1\n37658\t47019\tHampton\tTN\tCarter County\tH1\n37682\t47019\tMilligan college\tTN\tCarter County\tH1\n37694\t47019\tWatauga\tTN\tCarter County\tH1\n37601\t47019\tJohnson city\tTN\tCarter County\tH1\n37683\t47019\tMountain city\tTN\tCarter County\tH1\n37604\t47019\tJohnson city\tTN\tCarter County\tH1\n37643\t47019\tElizabethton\tTN\tCarter County\tH1\n37640\t47019\tButler\tTN\tCarter County\tH1\n37687\t47019\tRoan mountain\tTN\tCarter County\tH1\n37062\t47021\tFairview\tTN\tCheatham County\tH1\n37015\t47021\tAshland city\tTN\tCheatham County\tH1\n37043\t47021\tClarksville\tTN\tCheatham County\tH1\n37187\t47021\tWhite bluff\tTN\tCheatham County\tH1\n37035\t47021\tChapmansboro\tTN\tCheatham County\tH1\n37032\t47021\tCedar hill\tTN\tCheatham County\tH1\n37082\t47021\tKingston springs\tTN\tCheatham County\tH1\n37146\t47021\tPleasant view\tTN\tCheatham County\tH1\n37143\t47021\tPegram\tTN\tCheatham County\tH1\n37209\t47021\tNashville\tTN\tCheatham County\tH1\n37036\t47021\tCharlotte\tTN\tCheatham County\tH1\n37080\t47021\tJoelton\tTN\tCheatham County\tH1\n38371\t47023\tSardis\tTN\tChester County\tH1\n38352\t47023\tLuray\tTN\tChester County\tH1\n38366\t47023\tPinson\tTN\tChester County\tH1\n38356\t47023\tMedon\tTN\tChester County\tH1\n38313\t47023\tBeech bluff\tTN\tChester County\tH1\n38332\t47023\tEnville\tTN\tChester County\tH1\n38347\t47023\tJacks creek\tTN\tChester County\tH1\n38340\t47023\tHenderson\tTN\tChester County\tH1\n38334\t47023\tFinger\tTN\tChester County\tH1\n38368\t47023\tReagan\tTN\tChester County\tH1\n38315\t47023\tBethel springs\tTN\tChester County\tH1\n38359\t47023\tMilledgeville\tTN\tChester County\tH1\n38044\t47023\tHornsby\tTN\tChester County\tH1\n37851\t47025\tPruden\tTN\tClaiborne County\tH1\n37879\t47025\tTazewell\tTN\tClaiborne County\tH1\n37825\t47025\tNew tazewell\tTN\tClaiborne County\tH1\n37752\t47025\tHarrogate\tTN\tClaiborne County\tH1\n37869\t47025\tSneedville\tTN\tClaiborne County\tH1\n37715\t47025\tClairfield\tTN\tClaiborne County\tH1\n37724\t47025\tCumberland gap\tTN\tClaiborne County\tH1\n37870\t47025\tSpeedwell\tTN\tClaiborne County\tH1\n37881\t47025\tThorn hill\tTN\tClaiborne County\tH1\n37730\t47025\tEagan\tTN\tClaiborne County\tH1\n37707\t47025\tArthur\tTN\tClaiborne County\tH1\n38551\t47027\tCelina\tTN\tClay County\tH1\n38541\t47027\tAllons\tTN\tClay County\tH1\n38588\t47027\tWhitleyville\tTN\tClay County\tH1\n38575\t47027\tMoss\tTN\tClay County\tH1\n38568\t47027\tHilham\tTN\tClay County\tH1\n37150\t47027\tRed boiling springs\tTN\tClay County\tH1\n38573\t47027\tMonroe\tTN\tClay County\tH1\n37722\t47029\tCosby\tTN\tCocke County\tH1\n37821\t47029\tNewport\tTN\tCocke County\tH1\n37753\t47029\tHartford\tTN\tCocke County\tH1\n37743\t47029\tGreeneville\tTN\tCocke County\tH1\n37843\t47029\tParrottsville\tTN\tCocke County\tH1\n37818\t47029\tMosheim\tTN\tCocke County\tH1\n37727\t47029\tDel rio\tTN\tCocke County\tH1\n37713\t47029\tBybee\tTN\tCocke County\tH1\n37355\t47031\tManchester\tTN\tCoffee County\tH1\n37357\t47031\tMorrison\tTN\tCoffee County\tH1\n37389\t47031\tArnold afb\tTN\tCoffee County\tH1\n37366\t47031\tPelham\tTN\tCoffee County\tH1\n37183\t47031\tWartrace\tTN\tCoffee County\tH1\n37330\t47031\tEstill springs\tTN\tCoffee County\tH1\n37037\t47031\tChristiana\tTN\tCoffee County\tH1\n37388\t47031\tTullahoma\tTN\tCoffee County\tH1\n37026\t47031\tBradyville\tTN\tCoffee County\tH1\n37342\t47031\tHillsboro\tTN\tCoffee County\tH1\n37018\t47031\tBeechgrove\tTN\tCoffee County\tH1\n37382\t47031\tSummitville\tTN\tCoffee County\tH1\n37360\t47031\tNormandy\tTN\tCoffee County\tH1\n38006\t47033\tBells\tTN\tCrockett County\tH1\n38001\t47033\tAlamo\tTN\tCrockett County\tH1\n38336\t47033\tFruitvale\tTN\tCrockett County\tH1\n38040\t47033\tHalls\tTN\tCrockett County\tH1\n38050\t47033\tMaury city\tTN\tCrockett County\tH1\n38337\t47033\tGadsden\tTN\tCrockett County\tH1\n38034\t47033\tFriendship\tTN\tCrockett County\tH1\n38343\t47033\tHumboldt\tTN\tCrockett County\tH1\n38021\t47033\tCrockett mills\tTN\tCrockett County\tH1\n37381\t47035\tSpring city\tTN\tCumberland County\tH1\n37367\t47035\tPikeville\tTN\tCumberland County\tH1\n38583\t47035\tSparta\tTN\tCumberland County\tH1\n38572\t47035\tCrossville\tTN\tCumberland County\tH1\n38558\t47035\tCrossville\tTN\tCumberland County\tH1\n38571\t47035\tCrossville\tTN\tCumberland County\tH1\n38557\t47035\tCrossville\tTN\tCumberland County\tH1\n37337\t47035\tGrandview\tTN\tCumberland County\tH1\n37723\t47035\tCrab orchard\tTN\tCumberland County\tH1\n38578\t47035\tPleasant hill\tTN\tCumberland County\tH1\n37854\t47035\tRockwood\tTN\tCumberland County\tH1\n38574\t47035\tMonterey\tTN\tCumberland County\tH1\n38555\t47035\tCrossville\tTN\tCumberland County\tH1\n37211\t47037\tNashville\tTN\tDavidson County\tH6\n37208\t47037\tNashville\tTN\tDavidson County\tH6\n37218\t47037\tNashville\tTN\tDavidson County\tH6\n37243\t47037\tNashville\tTN\tDavidson County\tH6\n37086\t47037\tLa vergne\tTN\tDavidson County\tH6\n37115\t47037\tMadison\tTN\tDavidson County\tH6\n37232\t47037\tNashville\tTN\tDavidson County\tH6\n37202\t47037\tNashville\tTN\tDavidson County\tH6\n37242\t47037\tNashville\tTN\tDavidson County\tH6\n37250\t47037\tNashville\tTN\tDavidson County\tH6\n37246\t47037\tNashville\tTN\tDavidson County\tH6\n37013\t47037\tAntioch\tTN\tDavidson County\tH6\n37207\t47037\tNashville\tTN\tDavidson County\tH6\n37076\t47037\tHermitage\tTN\tDavidson County\tH6\n37073\t47037\tGreenbrier\tTN\tDavidson County\tH6\n37238\t47037\tNashville\tTN\tDavidson County\tH6\n37024\t47037\tBrentwood\tTN\tDavidson County\tH6\n37227\t47037\tNashville\tTN\tDavidson County\tH6\n37215\t47037\tNashville\tTN\tDavidson County\tH6\n37201\t47037\tNashville\tTN\tDavidson County\tH6\n37221\t47037\tNashville\tTN\tDavidson County\tH6\n37228\t47037\tNashville\tTN\tDavidson County\tH6\n37072\t47037\tGoodlettsville\tTN\tDavidson County\tH6\n37189\t47037\tWhites creek\tTN\tDavidson County\tH6\n37015\t47037\tAshland city\tTN\tDavidson County\tH6\n37203\t47037\tNashville\tTN\tDavidson County\tH6\n37206\t47037\tNashville\tTN\tDavidson County\tH6\n37216\t47037\tNashville\tTN\tDavidson County\tH6\n37122\t47037\tMount juliet\tTN\tDavidson County\tH6\n37135\t47037\tNolensville\tTN\tDavidson County\tH6\n37138\t47037\tOld hickory\tTN\tDavidson County\tH6\n37234\t47037\tNashville\tTN\tDavidson County\tH6\n37236\t47037\tNashville\tTN\tDavidson County\tH6\n37027\t47037\tBrentwood\tTN\tDavidson County\tH6\n37011\t47037\tAntioch\tTN\tDavidson County\tH6\n37204\t47037\tNashville\tTN\tDavidson County\tH6\n37214\t47037\tNashville\tTN\tDavidson County\tH6\n37219\t47037\tNashville\tTN\tDavidson County\tH6\n37070\t47037\tGoodlettsville\tTN\tDavidson County\tH6\n37220\t47037\tNashville\tTN\tDavidson County\tH6\n37143\t47037\tPegram\tTN\tDavidson County\tH6\n37064\t47037\tFranklin\tTN\tDavidson County\tH6\n37209\t47037\tNashville\tTN\tDavidson County\tH6\n37210\t47037\tNashville\tTN\tDavidson County\tH6\n37205\t47037\tNashville\tTN\tDavidson County\tH6\n37222\t47037\tNashville\tTN\tDavidson County\tH6\n37224\t47037\tNashville\tTN\tDavidson County\tH6\n37229\t47037\tNashville\tTN\tDavidson County\tH6\n37116\t47037\tMadison\tTN\tDavidson County\tH6\n37212\t47037\tNashville\tTN\tDavidson County\tH6\n37217\t47037\tNashville\tTN\tDavidson County\tH6\n37080\t47037\tJoelton\tTN\tDavidson County\tH6\n37213\t47037\tNashville\tTN\tDavidson County\tH6\n37240\t47037\tNashville\tTN\tDavidson County\tH6\n37235\t47037\tNashville\tTN\tDavidson County\tH6\n38371\t47039\tSardis\tTN\tDecatur County\tH1\n38311\t47039\tBath springs\tTN\tDecatur County\tH1\n38328\t47039\tDarden\tTN\tDecatur County\tH1\n38341\t47039\tHolladay\tTN\tDecatur County\tH1\n38329\t47039\tDecaturville\tTN\tDecatur County\tH1\n38388\t47039\tWildersville\tTN\tDecatur County\tH1\n38374\t47039\tScotts hill\tTN\tDecatur County\tH1\n38363\t47039\tParsons\tTN\tDecatur County\tH1\n38380\t47039\tSugar tree\tTN\tDecatur County\tH1\n37166\t47041\tSmithville\tTN\tDeKalb County\tH1\n38583\t47041\tSparta\tTN\tDeKalb County\tH1\n38567\t47041\tHickman\tTN\tDeKalb County\tH1\n37059\t47041\tDowelltown\tTN\tDeKalb County\tH1\n38569\t47041\tLancaster\tTN\tDeKalb County\tH1\n38582\t47041\tSilver point\tTN\tDeKalb County\tH1\n37095\t47041\tLiberty\tTN\tDeKalb County\tH1\n38581\t47041\tRock island\tTN\tDeKalb County\tH1\n37012\t47041\tAlexandria\tTN\tDeKalb County\tH1\n37184\t47041\tWatertown\tTN\tDeKalb County\tH1\n38548\t47041\tBuffalo valley\tTN\tDeKalb County\tH1\n38544\t47041\tBaxter\tTN\tDeKalb County\tH1\n37052\t47043\tCunningham\tTN\tDickson County\tH1\n37165\t47043\tSlayden\tTN\tDickson County\tH1\n37062\t47043\tFairview\tTN\tDickson County\tH1\n37187\t47043\tWhite bluff\tTN\tDickson County\tH1\n37181\t47043\tVanleer\tTN\tDickson County\tH1\n37029\t47043\tBurns\tTN\tDickson County\tH1\n37171\t47043\tSouthside\tTN\tDickson County\tH1\n37051\t47043\tCumberland furnace\tTN\tDickson County\tH1\n37056\t47043\tDickson\tTN\tDickson County\tH1\n37025\t47043\tBon aqua\tTN\tDickson County\tH1\n37036\t47043\tCharlotte\tTN\tDickson County\tH1\n37055\t47043\tDickson\tTN\tDickson County\tH1\n37101\t47043\tMc ewen\tTN\tDickson County\tH1\n38024\t47045\tDyersburg\tTN\tDyer County\tH1\n38007\t47045\tBogota\tTN\tDyer County\tH1\n38240\t47045\tObion\tTN\tDyer County\tH1\n38040\t47045\tHalls\tTN\tDyer County\tH1\n38047\t47045\tLenox\tTN\tDyer County\tH1\n38080\t47045\tRidgely\tTN\tDyer County\tH1\n38034\t47045\tFriendship\tTN\tDyer County\tH1\n38070\t47045\tTigrett\tTN\tDyer County\tH1\n38059\t47045\tNewbern\tTN\tDyer County\tH1\n38030\t47045\tFinley\tTN\tDyer County\tH1\n38025\t47045\tDyersburg\tTN\tDyer County\tH1\n38259\t47045\tTrimble\tTN\tDyer County\tH1\n38017\t47047\tCollierville\tTN\tFayette County\tH1\n38068\t47047\tSomerville\tTN\tFayette County\tH1\n38075\t47047\tWhiteville\tTN\tFayette County\tH1\n38036\t47047\tGallaway\tTN\tFayette County\tH1\n38057\t47047\tMoscow\tTN\tFayette County\tH1\n38069\t47047\tStanton\tTN\tFayette County\tH1\n38076\t47047\tWilliston\tTN\tFayette County\tH1\n38048\t47047\tMacon\tTN\tFayette County\tH1\n38060\t47047\tOakland\tTN\tFayette County\tH1\n38045\t47047\tLaconia\tTN\tFayette County\tH1\n38002\t47047\tArlington\tTN\tFayette County\tH1\n38039\t47047\tGrand junction\tTN\tFayette County\tH1\n38042\t47047\tHickory valley\tTN\tFayette County\tH1\n38046\t47047\tLa grange\tTN\tFayette County\tH1\n38049\t47047\tMason\tTN\tFayette County\tH1\n38028\t47047\tEads\tTN\tFayette County\tH1\n38066\t47047\tRossville\tTN\tFayette County\tH1\n38589\t47049\tWilder\tTN\tFentress County\tH1\n38565\t47049\tGrimsley\tTN\tFentress County\tH1\n38556\t47049\tJamestown\tTN\tFentress County\tH1\n38553\t47049\tClarkrange\tTN\tFentress County\tH1\n38504\t47049\tAllardt\tTN\tFentress County\tH1\n37726\t47049\tDeer lodge\tTN\tFentress County\tH1\n38574\t47049\tMonterey\tTN\tFentress County\tH1\n38549\t47049\tByrdstown\tTN\tFentress County\tH1\n38577\t47049\tPall mall\tTN\tFentress County\tH1\n38554\t47049\tCrawford\tTN\tFentress County\tH1\n37352\t47051\tLynchburg\tTN\tFranklin County\tH1\n37328\t47051\tElora\tTN\tFranklin County\tH1\n37376\t47051\tSherwood\tTN\tFranklin County\tH1\n37355\t47051\tManchester\tTN\tFranklin County\tH1\n37366\t47051\tPelham\tTN\tFranklin County\tH1\n37324\t47051\tDecherd\tTN\tFranklin County\tH1\n37330\t47051\tEstill springs\tTN\tFranklin County\tH1\n37388\t47051\tTullahoma\tTN\tFranklin County\tH1\n37318\t47051\tCowan\tTN\tFranklin County\tH1\n37398\t47051\tWinchester\tTN\tFranklin County\tH1\n37306\t47051\tBelvidere\tTN\tFranklin County\tH1\n37383\t47051\tSewanee\tTN\tFranklin County\tH1\n37345\t47051\tHuntland\tTN\tFranklin County\tH1\n37380\t47051\tSouth pittsburg\tTN\tFranklin County\tH1\n37375\t47051\tSewanee\tTN\tFranklin County\tH1\n37356\t47051\tMonteagle\tTN\tFranklin County\tH1\n37335\t47051\tFlintville\tTN\tFranklin County\tH1\n37160\t47051\tShelbyville\tTN\tFranklin County\tH1\n38220\t47053\tAtwood\tTN\tGibson County\tH1\n38358\t47053\tMilan\tTN\tGibson County\tH1\n38331\t47053\tEaton\tTN\tGibson County\tH1\n38369\t47053\tRutherford\tTN\tGibson County\tH1\n38330\t47053\tDyer\tTN\tGibson County\tH1\n38233\t47053\tKenton\tTN\tGibson County\tH1\n38348\t47053\tLavinia\tTN\tGibson County\tH1\n38316\t47053\tBradford\tTN\tGibson County\tH1\n38338\t47053\tGibson\tTN\tGibson County\tH1\n38382\t47053\tTrenton\tTN\tGibson County\tH1\n38346\t47053\tIdlewild\tTN\tGibson County\tH1\n38343\t47053\tHumboldt\tTN\tGibson County\tH1\n38059\t47053\tNewbern\tTN\tGibson County\tH1\n38355\t47053\tMedina\tTN\tGibson County\tH1\n38259\t47053\tTrimble\tTN\tGibson County\tH1\n38389\t47053\tYorkville\tTN\tGibson County\tH1\n38474\t47055\tMount pleasant\tTN\tGiles County\tH1\n38449\t47055\tArdmore\tTN\tGiles County\tH1\n37144\t47055\tPetersburg\tTN\tGiles County\tH1\n38456\t47055\t
